vi "LOAD data.vi"(11 "WFGraph Refnum":refnum<vi>) -> (2 "ok":bool, 3 "ng":bool)   [LabVIEW 2015]
uses:
  Galobal variable_TI.vi
  Project Setup/Globle Variable/GR_Servo.vi
panel:
  out "error out":errorcluster
  out "Boolean":bool
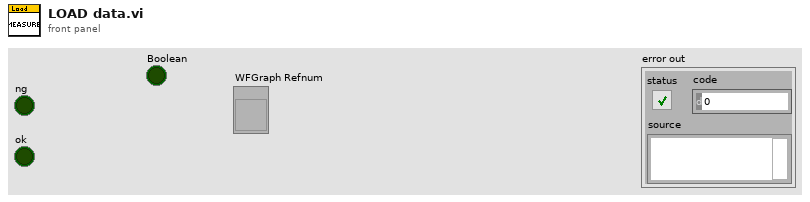
[diagram p1: front panel]
types:
  T1 = cluster{"Load Max(N)":dbl, "Load Min(N)":dbl, "Actuator1 max(mm)":dbl, "Actuator1min(mm)":dbl, "Actuator2 max(mm)":dbl, "Actuator2min(mm)":dbl, "Load Offset":dbl, "Model":string, "MIC Code":string}
  T2 = cluster{"Actuator1(mm)":dbl, "Actuator2(mm)":dbl, "Load(N)":dbl, "Actuator1":bool, "Actuator2":bool, "Load":bool}
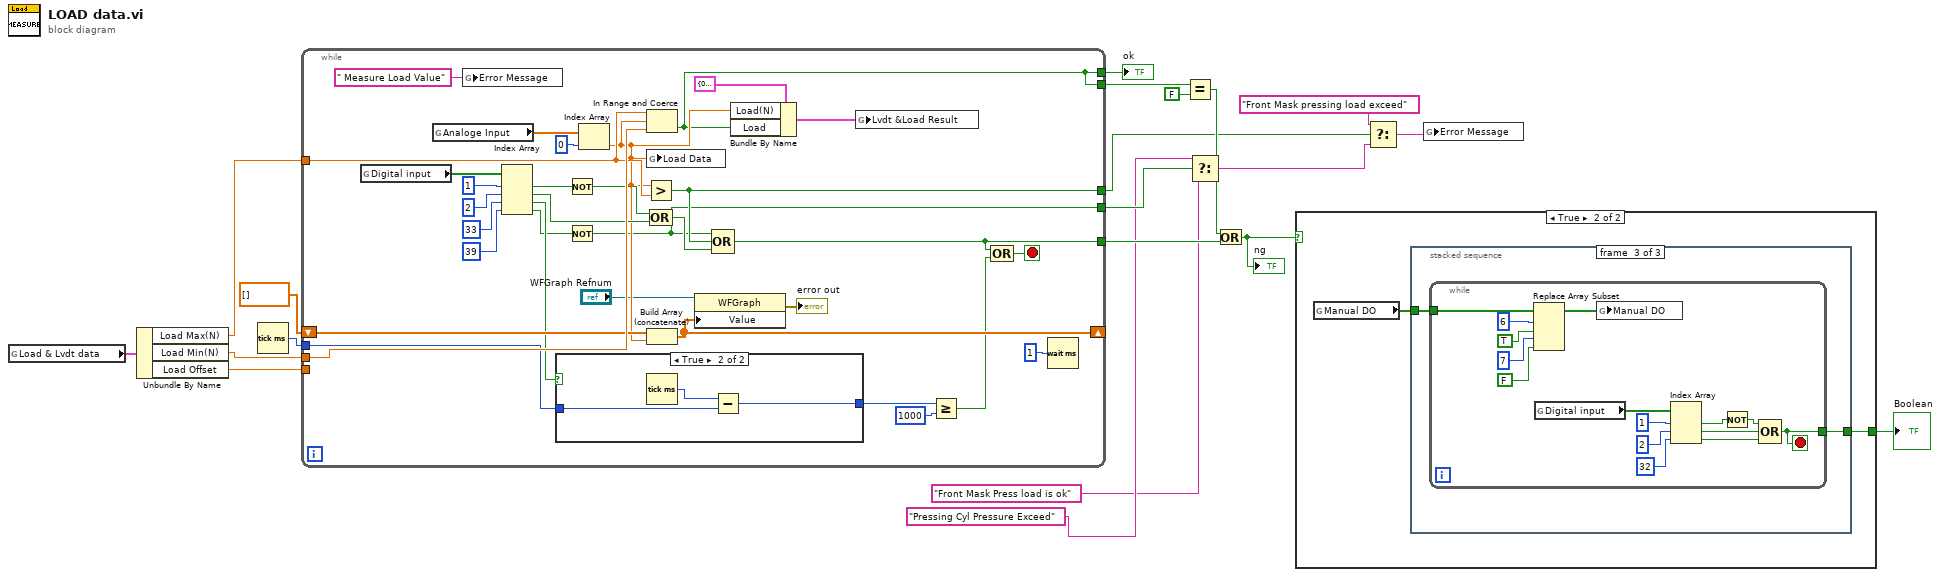
[diagram p0: block diagram]
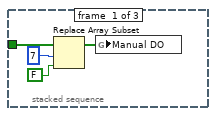
[diagram p3: hidden frame]
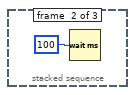
[diagram p4: hidden frame]
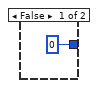
[diagram p5: hidden frame]
diagram:
  n1 = global read "Galobal variable_TI.vi" "Load & Lvdt data"() -> (w17:T1)
  n2 = Unbundle By Name(w17) -> ("Load Max(N)"=w18:dbl, "Load Min(N)"=w16:dbl, "Load Offset"=w19:dbl)
  n3 = Tick Count (ms)() -> (millisecond timer value=w10:u32)
  n4 = while {
    tunnel: w18 -> [w39]
    tunnel: w16 -> [w50]
    tunnel: w19 -> [_]
    tunnel: [w33] -> w20
    tunnel: [w32] -> w12
    tunnel: [w38] -> w6
    shift-right: [w34] -> _
    shift-left: dbl[] [] -> [w37]
    tunnel: [w33] -> w15
    tunnel: w10 -> [w29]
    tunnel: [w21] -> w4
    stop <- w43 stop-if-true
    n5 = global read "Galobal variable_TI.vi" "Digital input"() -> (w44:bool[])
    n6 = global read "Galobal variable_TI.vi" "Analoge Input"() -> (w52:dbl[])
    n7 = global write "GR_Servo.vi" "Error Message"(" Measure Load Value") -> ()
    n8 = Index Array(array=w44, index #1=1 ("index"), index #2=2 ("index"), index #3=33 ("index"), index #4=39 ("index")) -> (element #1=w48:bool, element #2=w45:bool, element #3=w30:bool, element #4=w25:bool)
    n9 = case shown="True" w30 {
      tunnel: w29 -> [_ w56]
      tunnel: [u32 0 w55] -> w28
      frame False {
      }
      frame True {
        n10 = Tick Count (ms)() -> (millisecond timer value=w57:u32)
        n11 = Subtract(x=w57, y=w56) -> (x-y=w55:u32)
      }
    }
    n12 = Not(x=w48) -> (.not. x?=w46:bool)
    n13 = Not(x=w25) -> (.not. x?=w21:bool)
    n14 = Index Array(array=w52, index=0) -> (element=w36:dbl)
    n15 = Greater?(x=w36, y=w39) -> (0:w38:bool)
    n16 = In Range and Coerce(upper limit=w39, x=w36, lower limit=w50) -> (In Range?=w33:bool)  [unwired: 1 out]
    n17 = global write "Galobal variable_TI.vi" "Load Data"(w36) -> ()
    n18 = Build Array (concatenate)(w37, w36) -> (w34:dbl[])
    n19 = Compound Arithmetic op=OR(w46, w45) -> (w22:bool)
    n20 = property class="WFGraph"(reference="WFGraph Refnum", "Value"=w34) -> (error out=→"error out":errorcluster)  [unwired: 1 in, 1 out]
    n21 = Compound Arithmetic op=OR(w21, w38, w22) -> (w32:bool)
    n22 = Bundle By Name(cluster=T2 {"Actuator1(mm)"=0.0, "Actuator2(mm)"=0.0, "Load(N)"=0.0, "Actuator1"=FALSE, "Actuator2"=FALSE, "Load"=FALSE} ("Lvdt &Load Result"), "Load(N)"=w36, "Load"=w33) -> (w40:T2)
    n23 = global write "Galobal variable_TI.vi" "Lvdt &Load Result"(w40) -> ()
    n24 = Greater Or Equal?(x=w28, y=u32 1000) -> (x >= y?=w24:bool)
    n25 = Compound Arithmetic op=OR(w32, w24) -> (w43:bool)
    n26 = Wait (ms)(milliseconds to wait=u32 1) -> ()  [unwired: 1 out]
  }
  "ok" <- w20
  n27 = Equal?(x=w15, y=FALSE) -> (x = y?=w13:bool)
  n28 = Select(t="Pressing Cyl Pressure Exceed" ("f"), s=w4, f="Front Mask Press load is ok") -> (s? t:f=w2:string)
  n29 = Or(x=w13, y=w12) -> (x .or. y?=w11:bool)
  "ng" <- w11
  n30 = case shown="True" w11 {
    tunnel: [_ w58] -> w9
    frame False {
    }
    frame True {
      n31 = global read "Galobal variable_TI.vi" "Manual DO"() -> (w59:bool[])
      n32 = stacked-sequence {
        tunnel: w59 -> [w63 _ w66]
        tunnel: [_ _ w65] -> w58
        frame #0 {
          n33 = Replace Array Subset(array=w63, new element=FALSE ("new element/subarray"), index=7) -> (w60:bool[])
          n34 = global write "Galobal variable_TI.vi" "Manual DO"(w60) -> ()
        }
        frame #1 {
          n35 = Wait (ms)(milliseconds to wait=u32 100) -> ()  [unwired: 1 out]
        }
        frame #2 {
          n36 = while {
            tunnel: w66 -> [w79]
            tunnel: [w69] -> w65
            stop <- w69 stop-if-true
            n37 = Replace Array Subset(array=w79, new element #1=TRUE ("new element/subarray"), index #1=6 ("index"), new element #2=FALSE ("new element/subarray"), index #2=7 ("index")) -> (w78:bool[])
            n38 = global read "Galobal variable_TI.vi" "Digital input"() -> (w76:bool[])
            n39 = global write "Galobal variable_TI.vi" "Manual DO"(w78) -> ()
            n40 = Index Array(array=w76, index #1=1 ("index"), index #2=2 ("index"), index #3=32 ("index")) -> (element #1=w73:bool, element #2=w71:bool, element #3=w70:bool)
            n41 = Not(x=w73) -> (.not. x?=w72:bool)
            n42 = Compound Arithmetic op=OR(w72, w71, w70) -> (w69:bool)
          }
        }
      }
    }
  }
  "Boolean" <- w9
  n43 = Select(t="Front Mask pressing load exceed", s=w6, f=w2) -> (s? t:f=w5:string)
  n44 = global write "GR_Servo.vi" "Error Message"(w5) -> ()
